vi "SetLiftSetpoint.vi"(11 "Buttons":bool[](array[boolean])) -> ()   [LabVIEW 2014]
uses:
  Gantry/GantryGlobals.vi
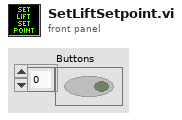
[diagram p1: front panel]
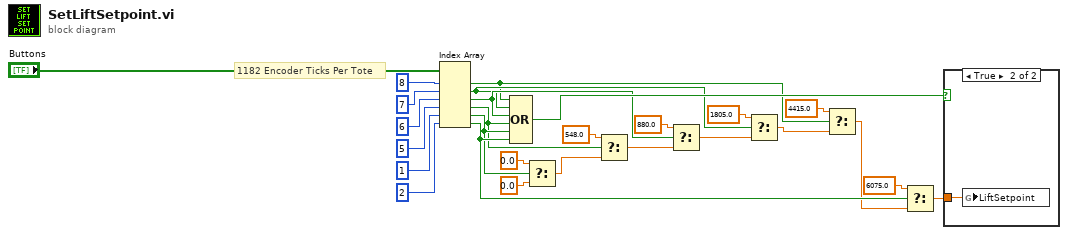
[diagram p0: block diagram]
diagram:
  # "1182 Encoder Ticks Per Tote"
  n1 = Index Array(array="Buttons", index #1=8 ("index"), index #2=7 ("index"), index #3=6 ("index"), index #4=5 ("index"), index #5=1 ("index"), index #6=2 ("index")) -> (element #1=w21:bool, element #2=w22:bool, element #3=w23:bool, element #4=w24:bool, element #5=w25:bool, element #6=w26:bool)
  n2 = Compound Arithmetic op=OR(w21, w22, w23, w24, w25, w26) -> (w27:bool)
  n3 = Select(t=0.0, s=w25, f=0.0) -> (s? t:f=w7:dbl)
  n4 = Select(t=548.0, s=w24, f=w7) -> (s? t:f=w10:dbl)
  n5 = Select(t=880.0, s=w23, f=w10) -> (s? t:f=w15:dbl)
  n6 = Select(t=1805.0, s=w22, f=w15) -> (s? t:f=w11:dbl)
  n7 = Select(t=4415.0, s=w21, f=w11) -> (s? t:f=w4:dbl)
  n8 = Select(t=6075.0, s=w26, f=w4) -> (s? t:f=w1:dbl)
  n9 = case shown="True" w27 {
    tunnel: w1 -> [_ w28]
    frame False {
    }
    frame True {
      n10 = global write "GantryGlobals.vi" "LiftSetpoint"(w28) -> ()
    }
  }
